vi "Panel.vi"(10 "Actor":refnum<class "Actor.lvclass">, 11 "Dev Actor Panel":refnum<class "Dev Actor Panel.lvclass">) -> ()   [LabVIEW 2021, in "Dev Actor Panel.lvclass"]
uses:
  Dev Actor Panel.lvclass
  src/LVCAM/LVCAM/Actor/Actor.lvclass
  Dev Actor Panel.lvclass/Dev Actor Panel.ctl
  Dev Actor/Dev Actor/Dev Actor.lvclass
  C:/git/jettl/src/LVCAM/LVCAM/Actor/Actor.lvclass
  src/LVCAM/Msgs/Actor Destroy/Actor Destroy Msg Strategy/Actor Destroy Msg Strategy.lvclass
  C:/git/jettl/src/LVCAM/LVCAM/Msg Strategy/Msg Strategy.lvclass
  src/LVCAM/Msgs/Actor Create/Actor Create Msg Strategy/Actor Create Msg Strategy.lvclass
panel:
  in  "Create Nested Actor":bool
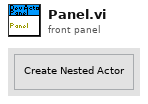
[diagram p1: front panel]
types:
  T1 = typedef "UEs.ctl" = cluster{"Teardown":refnum<user-event>}
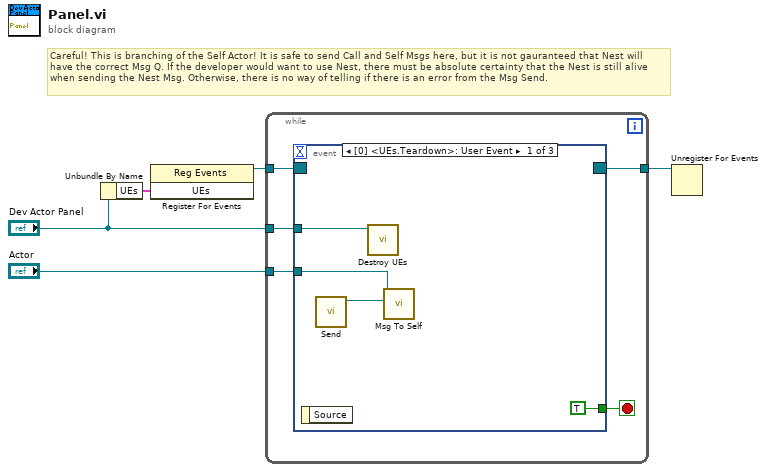
[diagram p0: block diagram]
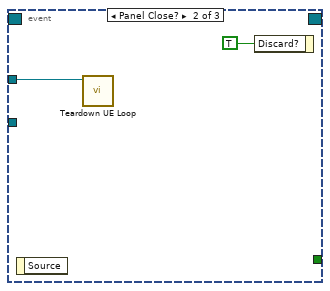
[diagram p2: hidden frame]
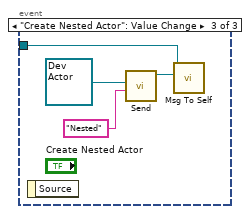
[diagram p3: hidden frame]
diagram:
  # "Careful! This is branching of the Self Actor! It is safe to send Call and Self Msgs here, but it is not gauranteed that Nest will have the correct Msg Q. If the developer would want to use Nest, there must be absolute certainty that the Nest is still alive when sending the Nest Msg. Otherwise, there is no way of telling if there is an error from the Msg Send."
  n1 = Unbundle By Name("Dev Actor Panel") -> ("UEs"=w3:T1)
  n2 = register-events ("Main Register for Events")(w3) -> (reference out=w4:refnum<event-registration>)  [unwired: 2 in, 1 out]
  n3 = while {
    tunnel: w4 -> [w10]
    tunnel: [w8] -> w5
    tunnel: "Actor" -> [w7]
    tunnel: "Dev Actor Panel" -> [w6]
    stop <- w9 stop-if-true
    n4 = event "UI Events" shown="[0] <UEs.Teardown>: User Event" {
      selector: w10 -> [_ _ _]
      dyn-events: [_ _ _] -> w8
      timeout: _ -> [_ _ _]
      tunnel: [TRUE _ _] -> w9
      tunnel: w7 -> [w12 _ w17]
      tunnel: w6 -> [w13 w15 _]
      event User Event {
        n5 = event-data() -> ()  [unwired: 1 in, 1 out]
        n6 = call "Send.vi"() -> ("Actor Destroy Msg Strategy out"=w11:refnum<class "Actor Destroy Msg Strategy.lvclass">)  [unwired: 11 in]
        n7 = call-dynamic "Destroy UEs.vi"("Dev Actor Panel in"=w13) -> ()  [unwired: 10 in, 1 out]
        n8 = call-dynamic "Msg To Self.vi"("Msg"=w11, "Actor in"=w12) -> ()  [unwired: 9 in, 1 out]
      }
      event Panel Close? {
        n9 = event-data() -> ()  [unwired: 1 in, 1 out]
        n10 = call-dynamic "Teardown UE Loop.vi"("Dev Actor Panel in"=w15) -> ()  [unwired: 10 in, 1 out]
        n11 = event-data("Discard?"=TRUE) -> ()  [unwired: 1 in, 1 out]
      }
      event "Create Nested Actor": Value Change {
        n12 = event-data() -> ()  [unwired: 1 in, 1 out]
        n13 = call "Send.vi"("Nested Alias"="Nested" ("Alias"), "Nested Actor"=refnum<class "Dev Actor.lvclass"> refnum ("ABD.lvlib:ABD.lvclass")) -> ("Actor Create Msg Strategy out"=w18:refnum<class "Actor Create Msg Strategy.lvclass">)  [unwired: 9 in]
        n14 = call-dynamic "Msg To Self.vi"("Msg"=w18, "Actor in"=w17) -> ()  [unwired: 9 in, 1 out]
      }
    }
  }
  n15 = Unregister For Events(event registration refnum=w5) -> ()  [unwired: 1 in, 1 out]
